vi "Main_Equip_Radiació.vi"() -> ()   [LabVIEW 2017]
uses:
  <vilib>/DAQmx/write.llb/DAQmx Write (Analog DBL 1Chan 1Samp).vi
  <vilib>/DAQmx/write.llb/DAQmx Write (Digital 1D Bool NChan 1Samp 1Line).vi
  <vilib>/DAQmx/read.llb/DAQmx Read (Digital 1D Bool NChan 1Samp 1Line).vi
  <vilib>/DAQmx/miscellaneous.llb/DAQmx Fill In Error Info.vi
panel:
  out "Primera":bool
  out "Factor":dbl
  out "T0":sgl caption="Temperatura" format="%.1f"
  in  "Tipo de Ensayo":enum32{"Calibración", "Ensayo A", "Ensayo B"}(radio)
  out "Nº Tests":u8 caption="Nº pruebas:"
  out "Columna":i32
  out "NMostres":dbl
  out "TablaFinal":dbl[][](array[numeric])
  in  "Consigna  (%)":dbl(slide) min=0.0 max=100.0 scale=0.0..100.0 scale format="%#_3g"
  in  "Poner Pantalla":bool
  in  "Disparo Pantalla":bool
  in  "HORNO":bool
  out "Pantalla retirada":bool
  out "Pantalla colocada":bool
  in  "Dades":dbl[](array[numeric])
  out "hardware name":string
  out "IndexSup":i32
  out "IndexInf":i32
  in  "Verifica":bool
  out "High Time":sgl format="%#_3g"
  out "Low Time":sgl format="%#_3g"
  in  "High Temp.":sgl
  in  "Low Temp.":sgl
  out "Temps":sgl caption="Tiempo" format="%.1f"
  out "Calibration result:":bool
  out "error out_USB":errorcluster
  out "Nom Sensor Temperatura":string
  in  "Guardar 24h":bool caption="Informe"
  out "Dies":u8 caption="NumDies"
  in  "Reset_AutoSave 24":bool
  in  "mT1":sgl caption="Temperatura_1" format="%.1f"
  out "Maxim":sgl
  in  "BtSalir":bool caption="Sortir"
  in  "Reset_AutoSave":bool
  in  "Nombre test:":string
  out "Gràfiques T-Temps":cluster{"Value":sgl[], "Value":sgl[]}[](graph)
  in  "Datos OK":bool
  out "DadesComplertes":sgl[](array[numeric])
  in  "Grafica_OK":bool=TRUE
  out "Tabla":sgl[][](array[numeric])
  in  "Registro OK":bool=TRUE
  in  "time out":bool
  in  "Reset_gráfica":bool
  in  "Reset_Time":bool
  in  "Tiempo_string":string[](array[string])
  out "Elapsed Time (s)":i32
  out "Ensayo activo":bool
  out "FSenseTara":sgl caption="Fuerza - N"
  in  "CaptadorF":u16(ring) caption="Unidades" items=["25kg"=5]
  in  "PendentLlum":sgl caption="Força" format="%.1f"
  out "FactorsUnitatsPendents_F":dbl[](array[numeric])
  out "ConversioUnitatsF":dbl[](array[numeric])=[1.0, 9.8756, 2.2]
  out "ArraiUnitats":cluster{"String":string, "Value":u16}[](array[cluster])=[{"String"="kg", "Value"=0}, {"String"="N", "Value"=1}, {"String"="g", "Value"=2}, {"String"="daN", "Value"=3}, {"String"="cN", "Value"=4}, {"String"="KN", "Value"=5}, {"String"="lb", "Value"=6}]
  out "Tara":sgl caption="Força" format="%.1f"
  out "Temperatura1":sgl caption="Temperatura" format="%.1f"
  out "PendentsT":sgl[](array[numeric])
  in  "Salir":bool caption="Sortir"
  in  "Ensayonuevo":bool caption="New Test"
  in  "Guardar":bool
  in  "Iniciar / Finalizar":bool=TRUE caption="Finalitzar prova"
  in  "UnidadesF":u16(ring) caption="Unidades" items=["kg", "N", "g"]
  in  "BtTaraPot":bool caption="TARA"
  # "sg"
  # "ºC"
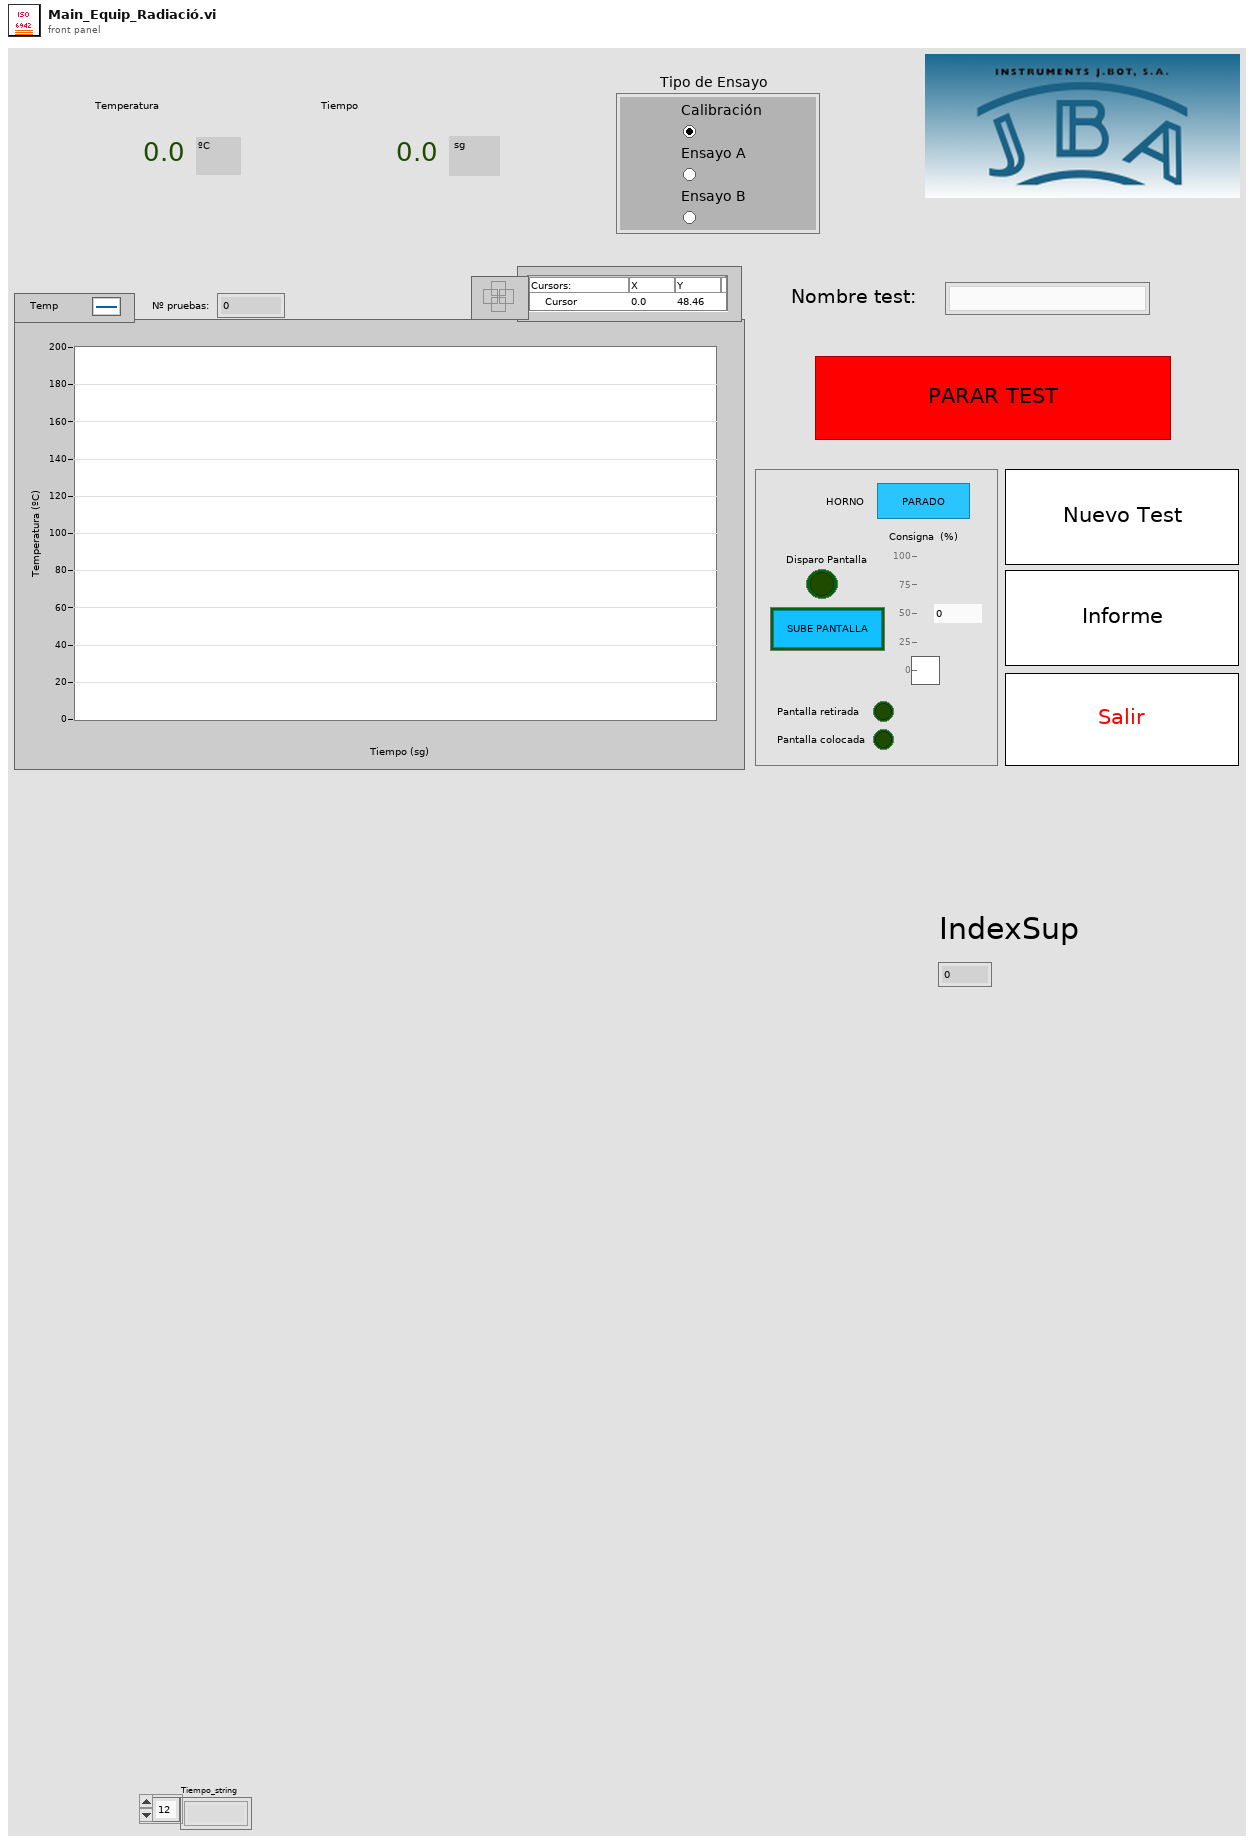
[diagram p1: front panel]
types:
  T1 = enum8{"Enabled", "Disabled", "Disabled and Grayed Out"}
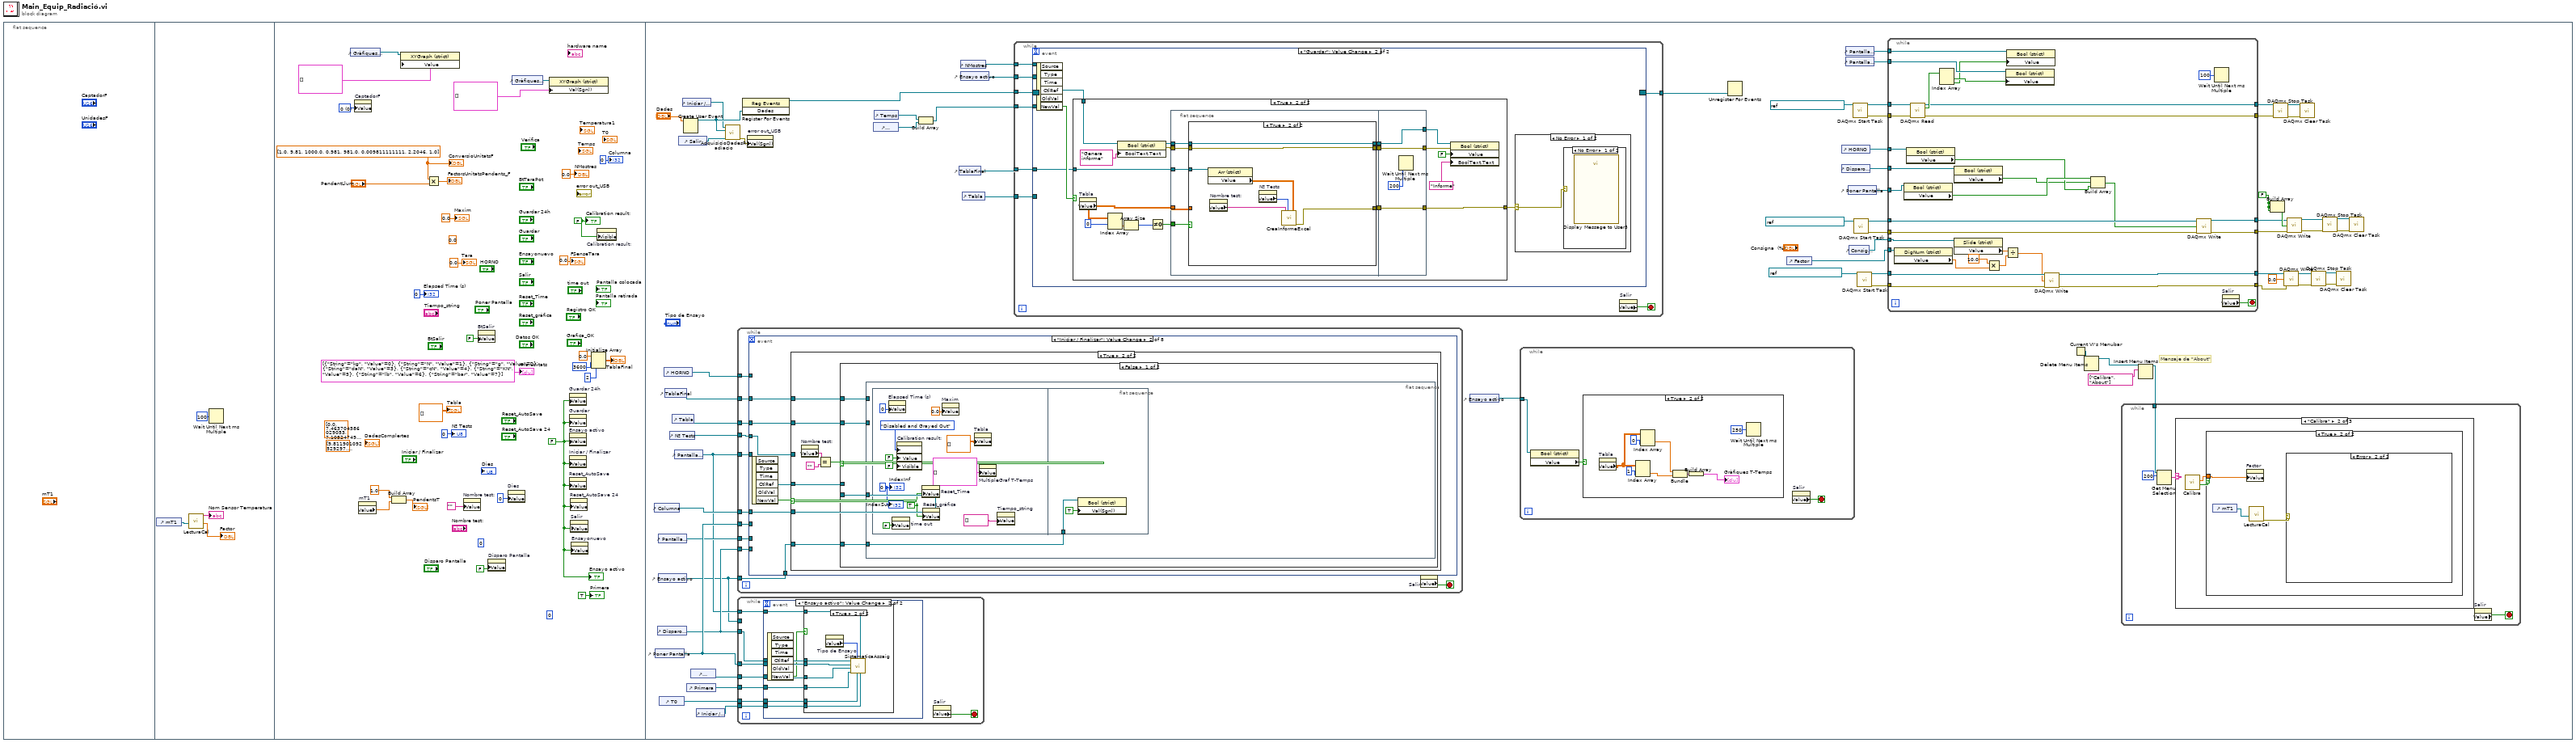
[diagram p0: block diagram]
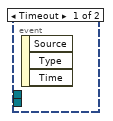
[diagram p2: hidden frame]
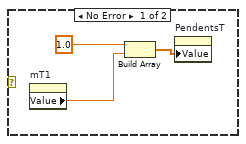
[diagram p6: hidden frame]
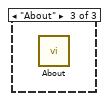
[diagram p7: hidden frame]
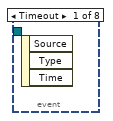
[diagram p9: hidden frame]
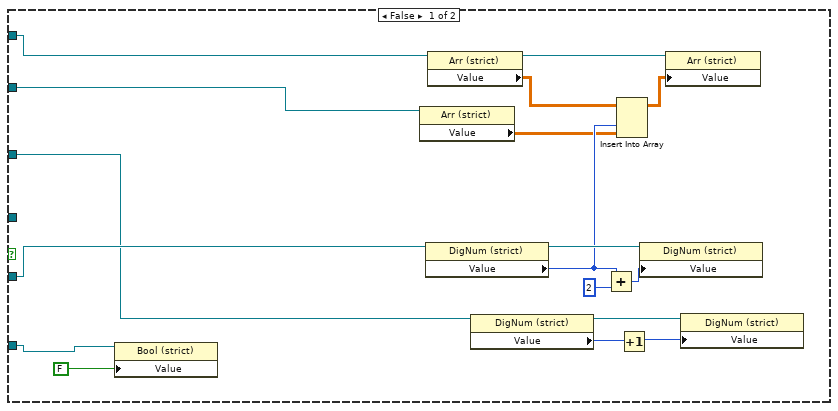
[diagram p10: hidden frame]
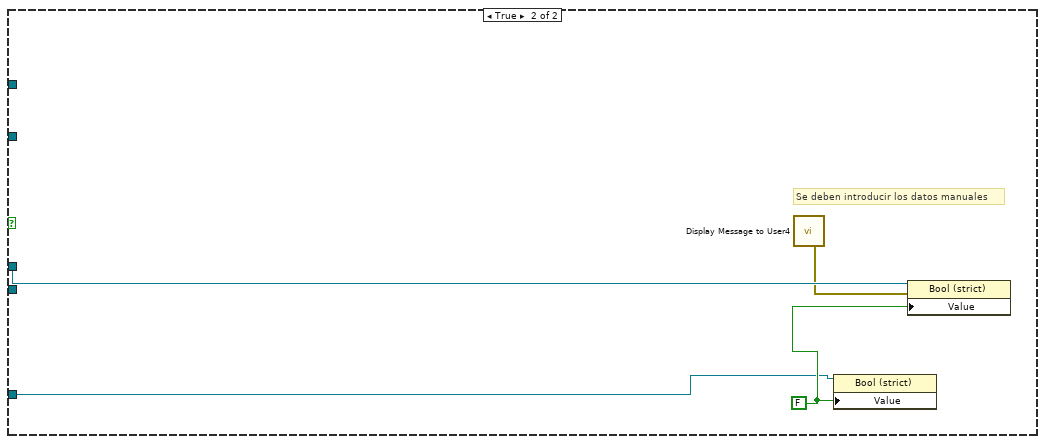
[diagram p11: hidden frame]
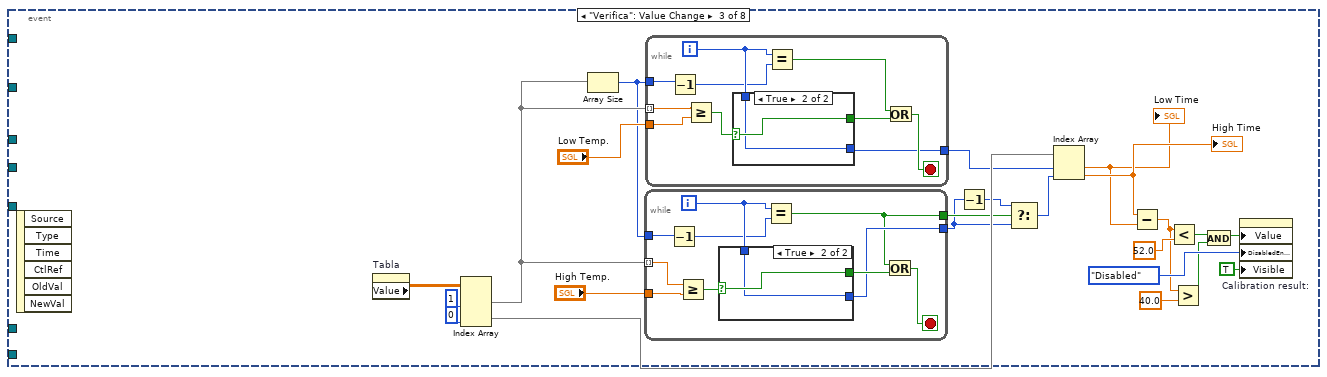
[diagram p12: hidden frame]
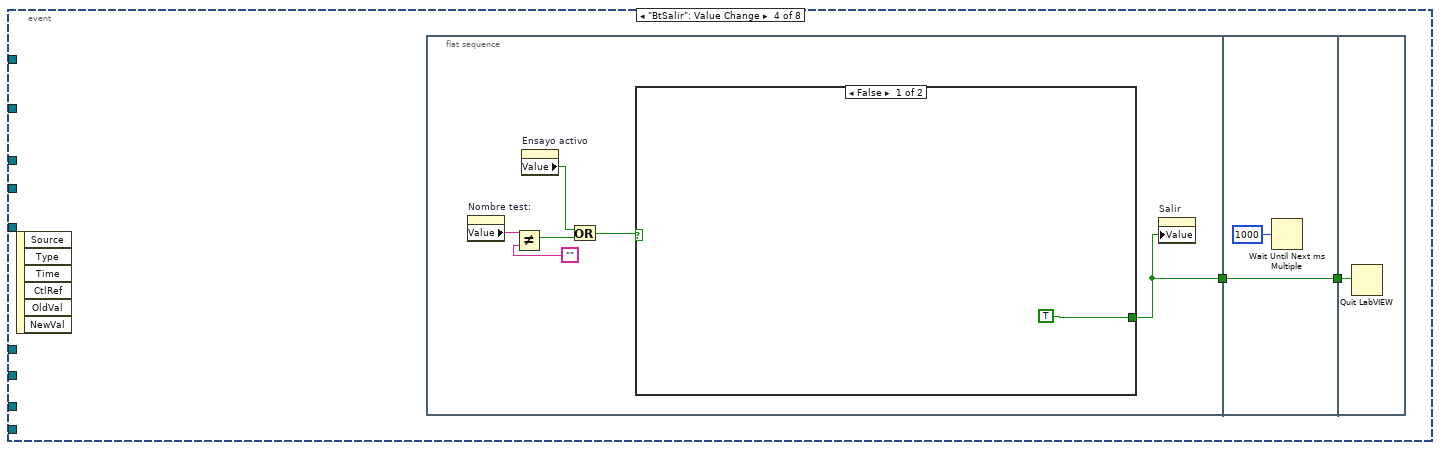
[diagram p15: hidden frame]
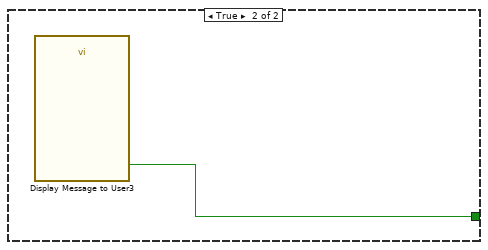
[diagram p16: hidden frame]
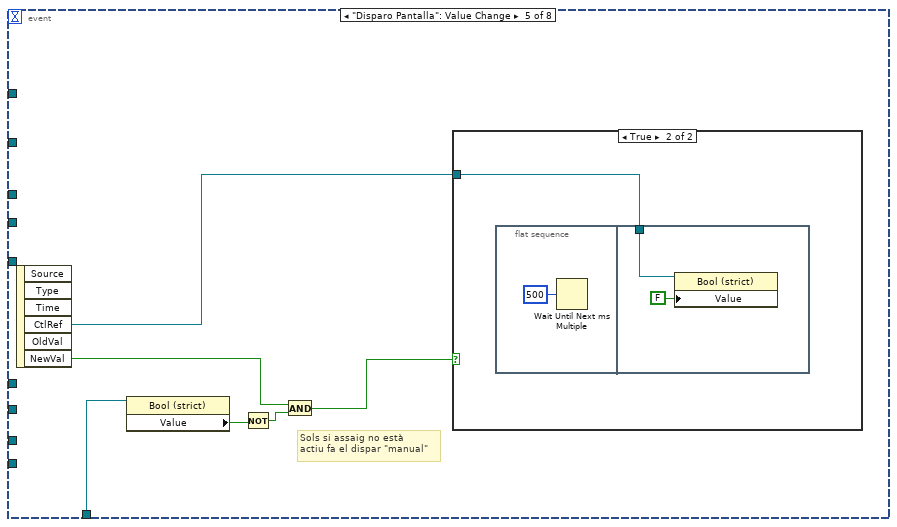
[diagram p17: hidden frame]
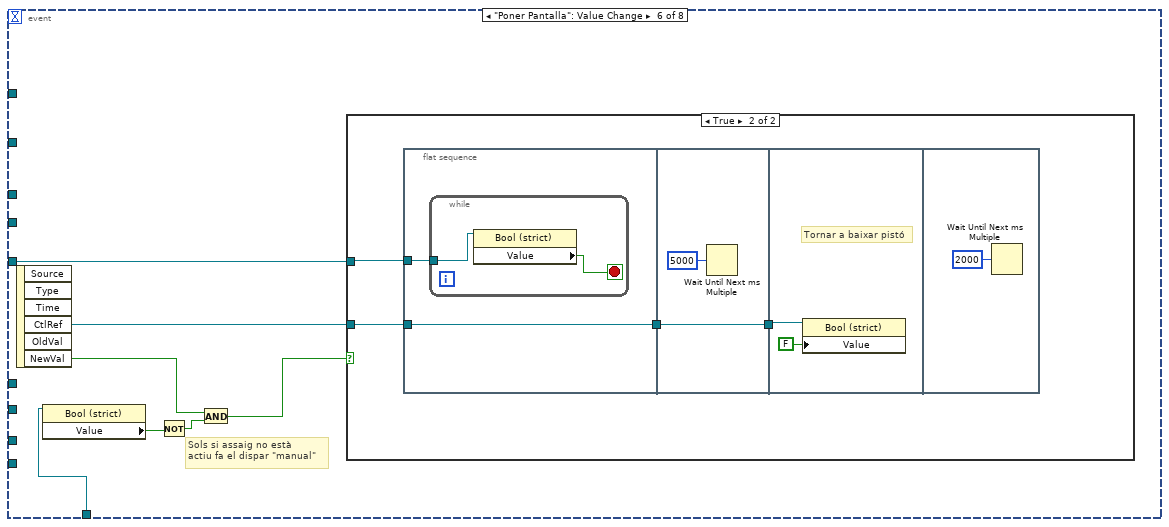
[diagram p19: hidden frame]
diagram:
  n1 = flat-sequence {
    frame #0 {
    }
    frame #1 {
      n2 = control-ref of="mT1"() -> (w2:refnum<vi>)
      n3 = call "LecturaCal.vi"("T1"=w2) -> ("Factor Potència"=→"Factor":dbl, "Nom Sensor Temperatura"=→"Nom Sensor Temperatura":string)  [unwired: 8 in, 1 out]
      n4 = Wait Until Next ms Multiple(millisecond multiple=u32 100) -> ()  [unwired: 1 out]
    }
    frame #2 {
      w18 = FALSE ("Resultat Assaig")
      (unwired) sgl[] [9.811901, 9.763803, 9.671529, 9.535354] ("DadesComplertes")
      (unwired) sgl[][] [[0.0, 7.4637046, 7.1052475, 6.7309566, 6.297442], [5.0, 2.5386999, 2.902987, 3.276568, 3.6958933], [10.0, 7.471229, 7.101099, 6.7181377, 6.2959595], [15.0, 2.5153666, 2.9171765, 3.291629, 3.679636], [20.0, 7.4759755, 7.089289, 6.711311, 6.298526]] ("Tabla")
      (unwired) u8 0 ("Durada assaig minuts")
      (unwired) u8 0 ("Durada assaig - hores:")
      w27 = u16 0 items=["0"] ("CaptadorF")
      (unwired) sgl 0.0 ("Fuerza")
      w6 = FALSE ("Ensayo activo")
      w34 = dbl[] [1.0, 9.81, 1000.0, 0.981, 981.0, 0.009811111111, 2.2046, 1.0]
      n5 = control-ref of="Gràfiques T-Temps"() -> (w20:refnum<vi>)
      n6 = property on="CaptadorF" class="Ring (strict)"("Value"=w27) -> ()  [unwired: 2 in, 2 out]
      n7 = property on="mT1" class="DigNum (strict)"() -> ("Value"=w7:sgl)  [unwired: 2 in, 2 out]
      n8 = Build Array(sgl 1.0 ("element"), w7) -> (→"PendentsT":sgl[])
      n9 = property class="XYGraph (strict)"(reference=w20, "Value"=cluster{"Value":sgl[], "Value":sgl[]}[] []) -> ()  [unwired: 1 in, 2 out]
      n10 = Multiply(x=w34, y="PendentLlum") -> (x*y=→"FactorsUnitatsPendents_F":dbl[])
      n11 = property on="Nombre test:" class="Str"("Value"="") -> ()  [unwired: 2 in, 2 out]
      n12 = property on="BtSalir" class="Bool (strict)"("Value"=FALSE ("BtSalir")) -> ()  [unwired: 2 in, 2 out]
      n13 = property on="Disparo Pantalla" class="Bool (strict)"("Value"=FALSE ("Quitar Pantalla")) -> ()  [unwired: 2 in, 2 out]
      n14 = property on="Dies" class="DigNum (strict)"("Value"=u8 0 ("NumDies")) -> ()  [unwired: 2 in, 2 out]
      n15 = control-ref of="Gràfiques T-Temps"() -> (w23:refnum<vi>)
      n16 = property class="XYGraph (strict)"(reference=w23, "Val(Sgnl)"=cluster{"Value":sgl[], "Value":sgl[]}[] [] ("Value")) -> ()  [unwired: 1 in, 2 out]
      n17 = property on="Guardar 24h" class="Bool (strict)"("Value"=w6) -> ()  [unwired: 2 in, 2 out]
      n18 = property on="Guardar" class="Bool (strict)"("Value"=w6) -> ()  [unwired: 2 in, 2 out]
      n19 = property on="Ensayo activo" class="Bool (strict)"("Value"=w6) -> ()  [unwired: 2 in, 2 out]
      n20 = property on="Iniciar / Finalizar" class="Bool (strict)"("Value"=w6) -> ()  [unwired: 2 in, 2 out]
      n21 = property on="Reset_AutoSave" class="Bool (strict)"("Value"=w6) -> ()  [unwired: 2 in, 2 out]
      n22 = property on="Reset_AutoSave 24" class="Bool (strict)"("Value"=w6) -> ()  [unwired: 2 in, 2 out]
      n23 = property on="Salir" class="Bool (strict)"("Value"=w6) -> ()  [unwired: 2 in, 2 out]
      n24 = property on="Ensayonuevo" class="Bool (strict)"("Value"=w6) -> ()  [unwired: 2 in, 2 out]
      n25 = Initialize Array(0.0 ("element"), 3600 ("dimension size"), 2 ("dimension size")) -> (→"TablaFinal":dbl[][])
      n26 = property on="Calibration result:" class="Bool (strict)"("Visible"=w18) -> ()  [unwired: 2 in, 2 out]
      "Tara" <- sgl 0.0 ("Tara")
      "ArraiUnitats" <- cluster{"String":string, "Value":u16}[] [{"String"="kg", "Value"=0}, {"String"="N", "Value"=1}, {"String"="g", "Value"=2}, {"String"="daN", "Value"=3}, {"String"="cN", "Value"=4}, {"String"="KN", "Value"=5}, {"String"="lb", "Value"=6}, {"String"="bar", "Value"=7}] ("Strings And Values [] 2")
      "ConversioUnitatsF" <- w34
      "FSenseTara" <- sgl 0.0 ("FSenseTara")
      "Elapsed Time (s)" <- 0 ("Elapsed Time (s)")
      "Tabla" <- sgl[][] [] ("Tabla")
      "Maxim" <- sgl 0.0 ("Maxim")
      "Calibration result:" <- w18
      "Ensayo activo" <- w6
      "NMostres" <- 0.0 ("NMostres")
      "Columna" <- 0 ("Columna")
      "Nº Tests" <- u8 0 ("Nº Tests")
      "Primera" <- TRUE ("Primera")
    }
    frame #3 {
      w47 = FALSE ("Value")
      # "Mensaje de \"About\""
      n27 = control-ref of="Columna"() -> (w64:refnum<vi>)
      n28 = control-ref of="Poner Pantalla"() -> (w55:refnum<vi>)
      n29 = control-ref of="Disparo Pantalla"() -> (w53:refnum<vi>)
      n30 = control-ref of="Pantalla retirada"() -> (w54:refnum<vi>)
      n31 = control-ref of="Ensayo activo"() -> (w48:refnum<vi>)
      n32 = control-ref of="T0"() -> (w57:refnum<vi>)
      n33 = control-ref of="HORNO"() -> (w59:refnum<vi>)
      n34 = control-ref of="TablaFinal"() -> (w65:refnum<vi>)
      n35 = control-ref of="Nº Tests"() -> (w62:refnum<vi>)
      n36 = control-ref of="Tabla"() -> (w63:refnum<vi>)
      n37 = control-ref of="Pantalla colocada"() -> (w51:refnum<vi>)
      n38 = control-ref of="Salir"() -> (w93:refnum<vi>)
      n39 = control-ref of="Iniciar / Finalizar"() -> (w89:refnum<vi>)
      n40 = Create User Event(user event datatype="Dades") -> (user event=w90:refnum<user-event>)  [unwired: 1 in, 1 out]
      n41 = control-ref of="Primera"() -> (w36:refnum<vi>)
      n42 = control-ref of="Temperatura1"() -> (w58:refnum<vi>)
      n43 = control-ref of="Iniciar / Finalizar"() -> (w52:refnum<vi>)
      n44 = call "AdquisicioDadesRadiacio.vi"("Stop"=w93, "EventDades"=w90, "AssaigActiu"=w89) -> ("error out"=w92:errorcluster)  [unwired: 8 in]
      n45 = while {
        tunnel: w65 -> [w193]
        tunnel: w64 -> [w192]
        tunnel: w63 -> [w191]
        tunnel: w62 -> [w190]
        tunnel: w59 -> [w189]
        tunnel: w51 -> [w188]
        tunnel: w55 -> [w187]
        tunnel: w54 -> [w186]
        tunnel: w53 -> [w185]
        tunnel: w48 -> [w184]
        stop <- w194 stop-if-true
        n46 = event shown="[1] \"Iniciar / Finalizar\": Value Change" {
          selector: _ -> [_ _ _ _ _ _ _ _]
          dyn-events: _ -> [_ _ _ _ _ _ _ _]
          timeout: _ -> [_ _ _ _ _ _ _ _]
          tunnel: w193 -> [_ w199 _ _ _ _ _ w343]
          tunnel: w192 -> [_ w198 _ _ _ _ _ w341]
          tunnel: w191 -> [_ w197 _ _ _ _ _ _]
          tunnel: w190 -> [_ w196 _ _ _ _ _ w345]
          tunnel: w189 -> [_ _ _ _ _ _ _ _]
          tunnel: w188 -> [_ _ _ _ _ w327 _ _]
          tunnel: w187 -> [_ _ _ _ _ _ _ _]
          tunnel: w186 -> [_ _ _ _ _ _ _ _]
          tunnel: w185 -> [_ _ _ _ _ _ _ _]
          tunnel: w184 -> [_ w195 _ _ w315 w323 _ _]
          event Timeout {
            n47 = event-data() -> ()  [unwired: 1 in, 3 out]
          }
          event "Iniciar / Finalizar": Value Change {
            n48 = event-data() -> ("CtlRef"=w200:refnum<vi>, "NewVal"=w201:bool)  [unwired: 1 in, 4 out]
            n49 = case shown="True" w201 {
              tunnel: w200 -> [_ w226]
              tunnel: w199 -> [w206 w225]
              tunnel: w198 -> [w209 w224]
              tunnel: w197 -> [w207 w223]
              tunnel: w196 -> [w208 _]
              tunnel: w195 -> [w203 w219]
              frame False {
                n50 = property class="Bool (strict)"(reference=w203, "Value"=FALSE ("Ensayo activo")) -> ()  [unwired: 1 in, 2 out]
                n51 = property class="Arr (strict)"(reference=w207) -> ("Value"=w213:sgl[][])  [unwired: 1 in, 2 out]
                n52 = property class="DigNum (strict)"(reference=w209) -> (reference out=w215:refnum<vi>, "Value"=w214:i32)  [unwired: 1 in, 1 out]
                n53 = property class="Arr (strict)"(reference=w206) -> (reference out=w205:refnum<vi>, "Value"=w211:dbl[][])  [unwired: 1 in, 1 out]
                n54 = property on="Property Node" class="DigNum (strict)"(reference=w208) -> (reference out=w204:refnum<vi>, "Value"=w217:u8)  [unwired: 1 in, 1 out]
                n55 = Add(x=w214, y=2) -> (x+y=w216:i32)
                n56 = Insert Into Array(array=w211, index (col)=w214, new element=w213) -> (w212:dbl[][])  [unwired: 1 in]
                n57 = Increment(x=w217) -> (x+1=w218:u8)
                n58 = property class="DigNum (strict)"(reference=w215, "Value"=w216) -> ()  [unwired: 1 in, 2 out]
                n59 = property class="Arr (strict)"(reference=w205, "Value"=w212) -> ()  [unwired: 1 in, 2 out]
                n60 = property on="Property Node" class="DigNum (strict)"(reference=w204, "Value"=w218) -> ()  [unwired: 1 in, 2 out]
              }
              frame True {
                n61 = property on="Nombre test:" class="Str"() -> ("Value"=w222:string)  [unwired: 2 in, 2 out]
                n62 = Equal?(x=w222, y="") -> (x = y?=w220:bool)
                n63 = case shown="False" w220 {
                  tunnel: w226 -> [_ w248]
                  tunnel: w225 -> [w230 _]
                  tunnel: w224 -> [w229 _]
                  tunnel: w223 -> [w228 _]
                  tunnel: w219 -> [w227 w245]
                  frame False {
                    n64 = flat-sequence {
                      tunnel: w228 -> [_]
                      tunnel: w229 -> [_]
                      tunnel: w230 -> [_]
                      tunnel: w227 -> [w231]
                      frame #0 {
                        n65 = flat-sequence {
                          tunnel: w231 -> [w244]
                          frame #0 {
                            w232 = 0 ("IndexInf")
                            w240 = TRUE ("Reset_Time")
                            n66 = property on="Elapsed Time (s)" class="DigNum (strict)"("Value"=0 ("Elapsed Time (s)")) -> ()  [unwired: 2 in, 2 out]
                            n67 = property on="time out" class="Bool (strict)"("Value"=FALSE ("time out")) -> ()  [unwired: 2 in, 2 out]
                            n68 = property on="Calibration result:" class="Bool (strict)"("DisabledEnum"=T1."Disabled and Grayed Out" ("Disabled"), "Value"=FALSE ("Resultat Assaig"), "Visible"=FALSE) -> ()  [unwired: 2 in, 2 out]
                            n69 = property on="Reset_Time" class="Bool (strict)"("Value"=w240) -> ()  [unwired: 2 in, 2 out]
                            n70 = property on="Reset_gráfica" class="Bool (strict)"("Value"=w240) -> ()  [unwired: 2 in, 2 out]
                            n71 = property on="Maxim" class="DigNum (strict)"("Value"=sgl 0.0 ("Maxim")) -> ()  [unwired: 2 in, 2 out]
                            n72 = property on="Tabla" class="Arr (strict)"("Value"=sgl[][] [] ("Tabla")) -> ()  [unwired: 2 in, 2 out]
                            n73 = property on="MultipleGraf T-Temps" class="XYGraph (strict)"("Value"=cluster{"Y":dbl[], "Y":dbl[]}[] []) -> ()  [unwired: 2 in, 2 out]
                            n74 = property on="Tiempo_string" class="Arr (strict)"("Value"=string[] [] ("Tiempo_string")) -> ()  [unwired: 2 in, 2 out]
                            "IndexSup" <- w232
                            "IndexInf" <- w232
                          }
                          frame #1 {
                            n75 = property class="Bool (strict)"(reference=w244, "Val(Sgnl)"=TRUE ("Iniciar assaig")) -> ()  [unwired: 1 in, 2 out]
                          }
                        }
                      }
                    }
                  }
                  frame True {
                    w246 = FALSE
                    # "Se deben introducir los datos manuales"
                    n76 = call "Display Message to User4"() -> ("error out"=w247:errorcluster)  [unwired: 10 in, 1 out]
                    n77 = property class="Bool (strict)"(reference=w245, "Value"=w246) -> ()  [unwired: 1 in, 2 out]
                    n78 = property class="Bool (strict)"(reference=w248, error in=w247, "Value"=w246) -> ()  [unwired: 2 out]
                  }
                }
              }
            }
          }
          event "Verifica": Value Change {
            n79 = event-data() -> ()  [unwired: 1 in, 6 out]
            n80 = property on="Tabla" class="Arr (strict)"() -> ("Value"=w271:sgl[][])  [unwired: 2 in, 2 out]
            n81 = Index Array(array=w271, index (col) #1=1 ("index (row)"), index (col) #2=0 ("index (row)")) -> (element #1=w262:sgl[], element #2=w259:sgl[])  [unwired: 2 in]
            n82 = Array Size(array=w262) -> (size(s)=w260:i32)
            n83 = while {
              tunnel: w262 -> [w281] mode=indexing
              tunnel: "High Temp." -> [w275]
              tunnel: w260 -> [w274]
              tunnel: [w273] -> w249
              tunnel: [w272] -> w252
              i -> [w279]
              stop <- w276 stop-if-true
              n84 = Decrement(x=w274) -> (x-1=w278:i32)
              n85 = Greater Or Equal?(x=w281, y=w275) -> (x >= y?=w280:bool)
              n86 = case shown="True" w280 {
                selector: w280 -> [w282 w284]
                tunnel: w279 -> [_ w283]
                tunnel: [w282 w284] -> w277
                tunnel: [_ w283] -> w273
                frame False {
                }
                frame True {
                }
              }
              n87 = Equal?(x=w279, y=w278) -> (x = y?=w272:bool)
              n88 = Or(x=w272, y=w277) -> (x .or. y?=w276:bool)
            }
            n89 = while {
              tunnel: w262 -> [w294] mode=indexing
              tunnel: "Low Temp." -> [w293]
              tunnel: w260 -> [w290]
              tunnel: [w285] -> w258
              i -> [w291]
              stop <- w286 stop-if-true
              n90 = Decrement(x=w290) -> (x-1=w289:i32)
              n91 = Greater Or Equal?(x=w294, y=w293) -> (x >= y?=w292:bool)
              n92 = case shown="True" w292 {
                selector: w292 -> [w295 w297]
                tunnel: w291 -> [_ w296]
                tunnel: [w295 w297] -> w287
                tunnel: [_ w296] -> w285
                frame False {
                }
                frame True {
                }
              }
              n93 = Equal?(x=w291, y=w289) -> (x = y?=w288:bool)
              n94 = Or(x=w288, y=w287) -> (x .or. y?=w286:bool)
            }
            n95 = Decrement(x=w249) -> (x-1=w250:i32)
            n96 = Select(t=w250, s=w252, f=w249) -> (s? t:f=w251:i32)
            n97 = Index Array(array=w259, index #1=w258, index #2=w251) -> (element #1=w266:sgl, element #2=w267:sgl)
            "Low Time" <- w266
            "High Time" <- w267
            n98 = Subtract(x=w267, y=w266) -> (x-y=w256:sgl)
            n99 = Less?(x=w256, y=sgl 52.0) -> (x < y?=w254:bool)
            n100 = Greater?(x=w256, y=40.0) -> (0:w253:bool)
            n101 = And(x=w254, y=w253) -> (x .and. y?=w255:bool)
            n102 = property on="Calibration result:" class="Bool (strict)"("Value"=w255, "DisabledEnum"=T1."Disabled" ("Disabled"), "Visible"=TRUE) -> ()  [unwired: 2 in, 2 out]
          }
          event "BtSalir": Value Change {
            n103 = event-data() -> ()  [unwired: 1 in, 6 out]
            n104 = flat-sequence {
              tunnel: [w305] -> w299
              tunnel: w299 -> [w309]
              tunnel: [w309] -> w298
              tunnel: w298 -> [w310]
              frame #0 {
                n105 = property on="Nombre test:" class="Str"() -> ("Value"=w304:string)  [unwired: 2 in, 2 out]
                n106 = Not Equal?(x=w304, y="") -> (x != y?=w300:bool)
                n107 = property on="Ensayo activo" class="Bool (strict)"() -> ("Value"=w301:bool)  [unwired: 2 in, 2 out]
                n108 = Or(x=w301, y=w300) -> (x .or. y?=w302:bool)
                n109 = case shown="False" w302 {
                  tunnel: [TRUE ("OK") w307] -> w305
                  frame False {
                  }
                  frame True {
                    n110 = call "Display Message to User3"() -> ("OK"=w307:bool)  [unwired: 10 in, 1 out]
                  }
                }
                n111 = property on="Salir" class="Bool (strict)"("Value"=w305) -> ()  [unwired: 2 in, 2 out]
              }
              frame #1 {
                n112 = Wait Until Next ms Multiple(millisecond multiple=u32 1000) -> ()  [unwired: 1 out]
              }
              frame #2 {
                n113 = Quit LabVIEW(quit? (T)=w310) -> ()
              }
            }
          }
          event "Disparo Pantalla": Value Change {
            # "Sols si assaig no està\nactiu fa el dispar \"manual\""
            n114 = event-data() -> ("CtlRef"=w316:refnum<vi>, "NewVal"=w312:bool)  [unwired: 1 in, 4 out]
            n115 = property class="Bool (strict)"(reference=w315) -> ("Value"=w314:bool)  [unwired: 1 in, 2 out]
            n116 = Not(x=w314) -> (.not. x?=w313:bool)
            n117 = And(x=w312, y=w313) -> (x .and. y?=w311:bool)
            n118 = case shown="True" w311 {
              tunnel: w316 -> [_ w317]
              frame False {
              }
              frame True {
                n119 = flat-sequence {
                  tunnel: w317 -> [w320]
                  frame #0 {
                    n120 = Wait Until Next ms Multiple(millisecond multiple=u32 500) -> ()  [unwired: 1 out]
                  }
                  frame #1 {
                    n121 = property class="Bool (strict)"(reference=w320, "Value"=FALSE) -> ()  [unwired: 1 in, 2 out]
                  }
                }
              }
            }
          }
          event "Poner Pantalla": Value Change {
            # "Sols si assaig no està\nactiu fa el dispar \"manual\""
            n122 = event-data() -> ("CtlRef"=w326:refnum<vi>, "NewVal"=w322:bool)  [unwired: 1 in, 4 out]
            n123 = property class="Bool (strict)"(reference=w323) -> ("Value"=w325:bool)  [unwired: 1 in, 2 out]
            n124 = Not(x=w325) -> (.not. x?=w324:bool)
            n125 = And(x=w322, y=w324) -> (x .and. y?=w321:bool)
            n126 = case shown="True" w321 {
              tunnel: w327 -> [_ w331]
              tunnel: w326 -> [_ w330]
              frame False {
              }
              frame True {
                n127 = flat-sequence {
                  tunnel: w331 -> [w333]
                  tunnel: w330 -> [w332]
                  tunnel: [w332] -> w329
                  tunnel: w329 -> [w336]
                  tunnel: [w336] -> w328
                  tunnel: w328 -> [w339]
                  frame #0 {
                    n128 = while {
                      tunnel: w333 -> [w335]
                      stop <- w334 stop-if-true
                      n129 = property class="Bool (strict)"(reference=w335) -> ("Value"=w334:bool)  [unwired: 1 in, 2 out]
                    }
                  }
                  frame #1 {
                    n130 = Wait Until Next ms Multiple(millisecond multiple=u32 5000) -> ()  [unwired: 1 out]
                  }
                  frame #2 {
                    # "Tornar a baixar pistó"
                    n131 = property class="Bool (strict)"(reference=w339, "Value"=FALSE) -> ()  [unwired: 1 in, 2 out]
                  }
                  frame #3 {
                    n132 = Wait Until Next ms Multiple(millisecond multiple=u32 2000) -> ()  [unwired: 1 out]
                  }
                }
              }
            }
          }
          event "error out_USB": Value Change {
            n133 = event-data() -> ()  [unwired: 1 in, 6 out]
            n134 = call "Display Message to User10"() -> ()  [unwired: 10 in, 2 out]
          }
          event "Ensayonuevo": Value Change {
            n135 = event-data() -> ("CtlRef"=w349:refnum<vi>, "NewVal"=w346:bool)  [unwired: 1 in, 4 out]
            n136 = property class="DigNum (strict)"(reference=w345) -> (reference out=w342:refnum<vi>, "Value"=w344:u8)  [unwired: 1 in, 1 out]
            n137 = Not Equal To 0?(x=w344) -> (x != 0?=w347:bool)
            n138 = And(x=w347, y=w346) -> (x .and. y?=w348:bool)
            n139 = case shown="True" w348 {
              tunnel: w349 -> [w353 w358]
              tunnel: [w353 w358] -> w350
              tunnel: [FALSE ("Value") FALSE ("Value")] -> w351
              tunnel: w343 -> [_ w356]
              tunnel: w342 -> [_ w355]
              tunnel: w341 -> [_ w354]
              frame False {
              }
              frame True {
                n140 = call "Display Message to User6"() -> ("Yes"=w359:bool)  [unwired: 10 in, 1 out]
                n141 = case shown="True" w359 {
                  tunnel: w356 -> [_ w366]
                  tunnel: w355 -> [_ w364]
                  tunnel: w354 -> [_ w362]
                  frame False {
                  }
                  frame True {
                    (unwired) "00:00:00" ("Tiempo transcurrido (hh:mm:ss)")
                    w371 = TRUE ("Reset_Time")
                    (unwired) cluster{"Value":sgl[], "Value":sgl[]} {"Value"=[], "Value"=[]} ("Grafica F-T")
                    n142 = property class="DigNum (strict)"(reference=w362, "Value"=0) -> ()  [unwired: 1 in, 2 out]
                    n143 = property class="Arr (strict)"(reference=w366, "Value"=dbl[][] []) -> ()  [unwired: 1 in, 2 out]
                    n144 = property class="DigNum (strict)"(reference=w364, "Value"=u8 0) -> ()  [unwired: 1 in, 2 out]
                    n145 = property on="Reset_Time" class="Bool (strict)"("Value"=w371) -> ()  [unwired: 2 in, 2 out]
                    n146 = property on="Reset_gráfica" class="Bool (strict)"("Value"=w371) -> ()  [unwired: 2 in, 2 out]
                    n147 = property on="Tiempo_string" class="Arr (strict)"("Value"=string[] [] ("Tiempo_string")) -> ()  [unwired: 2 in, 2 out]
                    n148 = property on="Nombre test:" class="Str"("Value"="") -> ()  [unwired: 2 in, 2 out]
                    n149 = property on="Tabla" class="Arr (strict)"("Value"=sgl[][] [] ("Tabla")) -> ()  [unwired: 2 in, 2 out]
                    n150 = property on="Gràfiques T-Temps" class="XYGraph (strict)"("Value"=cluster{"Y":dbl[], "Y":dbl[]}[] []) -> ()  [unwired: 2 in, 2 out]
                    n151 = property on="Primera" class="Bool (strict)"("Value"=TRUE ("Primera")) -> ()  [unwired: 2 in, 2 out]
                    n152 = property on="Elapsed Time (s)" class="DigNum (strict)"("Value"=0 ("Elapsed Time (s)")) -> ()  [unwired: 2 in, 2 out]
                    n153 = property on="time out" class="Bool (strict)"("Value"=FALSE ("time out")) -> ()  [unwired: 2 in, 2 out]
                    n154 = property on="Maxim" class="DigNum (strict)"("Value"=sgl 0.0 ("Maxim")) -> ()  [unwired: 2 in, 2 out]
                  }
                }
              }
            }
            n155 = property class="Bool (strict)"(reference=w350, "Value"=w351) -> ()  [unwired: 1 in, 2 out]
          }
        }
        n156 = property on="Salir" class="Bool (strict)"() -> ("Value"=w194:bool)  [unwired: 2 in, 2 out]
      }
      n157 = while {
        tunnel: w58 -> [w111]
        tunnel: w57 -> [w110]
        tunnel: w53 -> [w109]
        tunnel: w55 -> [w108]
        tunnel: w48 -> [_]
        tunnel: w52 -> [w106]
        tunnel: w51 -> [w105]
        tunnel: w36 -> [w104]
        stop <- w107 stop-if-true
        n158 = event shown="[1] \"Ensayo activo\": Value Change" {
          selector: _ -> [_ _]
          dyn-events: _ -> [_ _]
          timeout: _ -> [_ _]
          tunnel: w111 -> [_ w119]
          tunnel: w110 -> [_ w118]
          tunnel: w109 -> [_ w117]
          tunnel: w108 -> [_ w116]
          tunnel: w106 -> [_ w115]
          tunnel: w105 -> [_ w114]
          tunnel: w104 -> [_ w113]
          event Timeout {
            n159 = event-data() -> ()  [unwired: 1 in, 3 out]
          }
          event "Ensayo activo": Value Change {
            n160 = event-data() -> ("NewVal"=w112:bool)  [unwired: 1 in, 5 out]
            n161 = case shown="True" w112 {
              tunnel: w119 -> [_ w126]
              tunnel: w118 -> [_ w125]
              tunnel: w117 -> [_ w124]
              tunnel: w116 -> [_ w123]
              tunnel: w115 -> [_ w122]
              tunnel: w114 -> [_ w121]
              tunnel: w113 -> [_ w120]
              frame False {
              }
              frame True {
                n162 = property on="Tipo de Ensayo" class="RadioBtnsControl (strict)"() -> ("Value"=w127:enum32{"Calibración", "Ensayo A", "Ensayo B"})  [unwired: 2 in, 2 out]
                n163 = call "SistematicaAssaig.vi"("Iniciar/Finalitzar"=w122, "PantallaColocada"=w121, "T0"=w125, "Value"=w127, "Primera"=w120, "Temperatura1"=w126, "Poner Pantalla"=w123, "DisparoPantalla"=w124) -> ()  [unwired: 4 in]
              }
            }
          }
        }
        n164 = property on="Salir" class="Bool (strict)"() -> ("Value"=w107:bool)  [unwired: 2 in, 2 out]
      }
      n165 = register-events(w90) -> (reference out=w102:refnum<event-registration>)  [unwired: 2 in, 1 out]
      n166 = property on="error out_USB" class="Clust (strict)"("Val(Sgnl)"=w92) -> ()  [unwired: 2 in, 2 out]
      n167 = control-ref of="Temperatura1"() -> (w94:refnum<vi>)
      n168 = control-ref of="Temps"() -> (w95:refnum<vi>)
      n169 = Build Array(w95, w94) -> (w97:refnum<vi>[])
      n170 = control-ref of="TablaFinal"() -> (w61:refnum<vi>)
      n171 = control-ref of="NMostres"() -> (w66:refnum<vi>)
      n172 = control-ref of="Ensayo activo"() -> (w96:refnum<vi>)
      n173 = control-ref of="Tabla"() -> (w60:refnum<vi>)
      n174 = while {
        tunnel: w102 -> [w382]
        tunnel: [w381] -> w103
        tunnel: w97 -> [w379]
        tunnel: w96 -> [w378]
        tunnel: w66 -> [w377]
        tunnel: w61 -> [w376]
        tunnel: w60 -> [w375]
        stop <- w380 stop-if-true
        n175 = event shown="[1] \"Guardar\": Value Change" {
          selector: w382 -> [_ _]
          dyn-events: [_ _] -> w381
          timeout: _ -> [_ _]
          tunnel: w379 -> [w389 _]
          tunnel: w378 -> [w388 _]
          tunnel: w377 -> [w384 _]
          tunnel: w376 -> [_ w404]
          tunnel: w375 -> [w383 _]
          event User Event {
            n176 = event-data() -> ("Dades"=w385:dbl[])  [unwired: 1 in, 4 out]
            n177 = property on="PendentsT" class="Arr (strict)"() -> ("Value"=w390:sgl[])  [unwired: 2 in, 2 out]
            n178 = Multiply(x=w385, y=w390) -> (x*y=w386:dbl[])
            n179 = for {
              tunnel: w389 -> [w392] mode=indexing
              tunnel: w386 -> [w393] mode=indexing
              # "Precisió 2 i 1"
              n180 = property class="DigNum (strict)"(reference=w392, "Value"=w393, "Precision"=u8 1 ("Display Format:Precision")) -> ()  [unwired: 1 in, 2 out]
            }
            n181 = property class="Bool (strict)"(reference=w388) -> ("Value"=w387:bool)  [unwired: 1 in, 2 out]
            n182 = case shown="True" w387 {
              tunnel: w386 -> [_ w394]
              tunnel: w384 -> [_ w403]
              tunnel: w383 -> [_ w398]
              frame False {
              }
              frame True {
                n183 = property class="DigNum (strict)"(reference=w403) -> (reference out=w402:refnum<vi>, error out=w401:errorcluster, "Value"=w400:dbl)  [unwired: 1 in]
                n184 = property class="Arr (strict)"(reference=w398) -> (reference out=w397:refnum<vi>, "Value"=w396:sgl[][])  [unwired: 1 in, 1 out]
                n185 = Build Array (concatenate)(w396, w394) -> (w395:dbl[][])
                n186 = Increment(x=w400) -> (x+1=w399:dbl)
                n187 = property class="DigNum (strict)"(reference=w402, error in=w401, "Value"=w399) -> ()  [unwired: 2 out]
                n188 = property class="Arr (strict)"(reference=w397, "Value"=w395) -> ()  [unwired: 1 in, 2 out]
              }
            }
          }
          event "Guardar": Value Change {
            n189 = event-data() -> ("CtlRef"=w405:refnum<vi>, "NewVal"=w407:bool)  [unwired: 1 in, 4 out]
            n190 = case shown="True" w407 {
              tunnel: [errorcluster {"status"=FALSE, "code"=0, "source"=""} ("error out") w428] -> w406
              tunnel: w405 -> [_ w418]
              tunnel: w404 -> [_ w411]
              frame False {
              }
              frame True {
                n191 = property on="Tabla" class="Arr (strict)"() -> ("Value"=w412:sgl[][])  [unwired: 2 in, 2 out]
                n192 = Index Array(array=w412, index (row)=0) -> (element=w426:sgl[])  [unwired: 1 in]
                n193 = property class="Bool (strict)"(reference=w418, "BoolText.Text"="Genera informe" ("Boolean Text.Text")) -> (reference out=w417:refnum<vi>, error out=w413:errorcluster)  [unwired: 1 in]
                n194 = Array Size(array=w426) -> (size(s)=w414:i32)
                n195 = Not Equal To 0?(x=w414) -> (x != 0?=w425:bool)
                n196 = flat-sequence {
                  tunnel: w412 -> [w435]
                  tunnel: w425 -> [w434]
                  tunnel: w417 -> [w432]
                  tunnel: [w436] -> w421
                  tunnel: [w433] -> w420
                  tunnel: [w431] -> w419
                  tunnel: w413 -> [w430]
                  tunnel: w411 -> [w429]
                  tunnel: [w448] -> w423
                  tunnel: [w449] -> w424
                  tunnel: [w450] -> w428
                  tunnel: w421 -> [w450]
                  tunnel: w420 -> [w449]
                  tunnel: w419 -> [w448]
                  frame #0 {
                    n197 = case shown="True" w434 {
                      tunnel: [errorcluster {"status"=TRUE, "code"=0, "source"=""} ("error out") w444] -> w436
                      tunnel: w435 -> [_ _]
                      tunnel: [w438 w443] -> w433
                      tunnel: w432 -> [w437 w446]
                      tunnel: [w437 w446] -> w431
                      tunnel: w430 -> [_ w443]
                      tunnel: w429 -> [_ w440]
                      frame False {
                        n198 = call "Display Message to User8"() -> ("error out"=w438:errorcluster)  [unwired: 10 in, 1 out]
                      }
                      frame True {
                        n199 = property class="Arr (strict)"(reference=w440) -> ("Value"=w442:dbl[][])  [unwired: 1 in, 2 out]
                        n200 = property on="Nombre test:" class="Str"() -> ("Value"=w445:string)  [unwired: 2 in, 2 out]
                        n201 = property on="Nº Tests" class="DigNum (strict)"() -> ("Value"=w441:u8)  [unwired: 2 in, 2 out]
                        n202 = call "CreaInformeExcel.vi"("Nom Assaig"=w445, "NºTests"=w441, "Tabla"=w442) -> ("error out"=w444:errorcluster)  [unwired: 15 in, 1 out]
                      }
                    }
                  }
                  frame #1 {
                    n203 = Wait Until Next ms Multiple(millisecond multiple=u32 200 ("milliseconds to wait")) -> ()  [unwired: 1 out]
                  }
                }
                n204 = property class="Bool (strict)"(reference=w423, error in=w424, "Value"=FALSE, "BoolText.Text"="Informe" ("Boolean Text.Text")) -> ()  [unwired: 2 out]
              }
            }
            n205 = case shown="No Error" w406 {
              selector: w406 -> [w408 _]
              frame No Error {
                n206 = case shown="No Error" w408 {
                  frame No Error {
                    n207 = call "Display Message to User5"() -> ()  [unwired: 10 in, 2 out]
                  }
                  frame Error {
                    n208 = property on="Reset_AutoSave" class="Bool (strict)"("Value"=FALSE ("Reset_AutoSave")) -> ()  [unwired: 2 in, 2 out]
                  }
                }
              }
              frame Error {
              }
            }
          }
        }
        n209 = property on="Salir" class="Bool (strict)"() -> ("Value"=w380:bool)  [unwired: 2 in, 2 out]
      }
      n210 = control-ref of="Ensayo activo"() -> (w56:refnum<vi>)
      n211 = while {
        tunnel: w56 -> [w174]
        stop <- w175 stop-if-true
        n212 = property class="Bool (strict)"(reference=w174) -> ("Value"=w173:bool)  [unwired: 1 in, 2 out]
        n213 = case shown="True" w173 {
          frame False {
          }
          frame True {
            n214 = property on="Tabla" class="Arr (strict)"() -> ("Value"=w179:sgl[][])  [unwired: 2 in, 2 out]
            n215 = Index Array(array=w179, index (col)=1 ("index")) -> (element=w178:sgl[])  [unwired: 1 in]
            n216 = Index Array(array=w179, index (col)=0 ("index (row)")) -> (element=w177:sgl[])  [unwired: 1 in]
            n217 = Bundle("Value"=w177, "Value"=w178) -> (w183:cluster{"Value":sgl[], "Value":sgl[]})  [unwired: 1 in]
            n218 = Build Array(w183) -> (→"Gràfiques T-Temps":cluster{"Value":sgl[], "Value":sgl[]}[])
            n219 = Wait Until Next ms Multiple(millisecond multiple=u32 250) -> ()  [unwired: 1 out]
          }
        }
        n220 = property on="Salir" class="Bool (strict)"() -> ("Value"=w175:bool)  [unwired: 2 in, 2 out]
      }
      n221 = Unregister For Events(event registration refnum=w103) -> ()  [unwired: 1 in, 1 out]
      n222 = control-ref of="Factor"() -> (w50:refnum<vi>)
      n223 = control-ref of="HORNO"() -> (w76:refnum<vi>)
      n224 = control-ref of="Disparo Pantalla"() -> (w75:refnum<vi>)
      n225 = control-ref of="Pantalla colocada"() -> (w81:refnum<vi>)
      n226 = control-ref of="Pantalla retirada"() -> (w80:refnum<vi>)
      n227 = control-ref of="Poner Pantalla"() -> (w74:refnum<vi>)
      n228 = control-ref of="Consigna  (%)"() -> (w71:refnum<vi>)
      n229 = call <vilib>:"DAQmx Start Task.vi"("task/channels in"=refnum<k21> "USB_Equip_Radiacio_DIn") -> ("task out"=w86:refnum<k21>, "error out"=w70:errorcluster)  [unwired: 13 in]
      n230 = call <vilib>:"DAQmx Start Task.vi"("task/channels in"=refnum<k21> "USB_Equip_Radiacio_DOut") -> ("task out"=w85:refnum<k21>, "error out"=w49:errorcluster)  [unwired: 13 in]
      n231 = call <vilib>:"DAQmx Start Task.vi"("task/channels in"=refnum<k21> "USB_Equip_Radiacio_AO") -> ("task out"=w72:refnum<k21>, "error out"=w69:errorcluster)  [unwired: 13 in]
      n232 = while {
        tunnel: w86 -> [w159]
        tunnel: w85 -> [w154]
        tunnel: [w157] -> w84
        tunnel: w81 -> [w156]
        tunnel: w80 -> [w155]
        tunnel: [w153] -> w44
        tunnel: [w152] -> w77
        tunnel: [w151] -> w43
        tunnel: w76 -> [w150]
        tunnel: w75 -> [w149]
        tunnel: w74 -> [w148]
        tunnel: w72 -> [w147]
        tunnel: w71 -> [w146]
        tunnel: w70 -> [w145]
        tunnel: w69 -> [w144]
        tunnel: [w143] -> w40
        tunnel: [w142] -> w39
        tunnel: w50 -> [w131]
        tunnel: w49 -> [w129]
        stop <- w160 stop-if-true
        n233 = property class="DigNum (strict)"(reference=w131) -> ("Value"=w130:dbl)  [unwired: 1 in, 2 out]
        n234 = property class="Bool (strict)"(reference=w148) -> ("Value"=w141:bool)  [unwired: 1 in, 2 out]
        n235 = property class="Bool (strict)"(reference=w150) -> ("Value"=w136:bool)  [unwired: 1 in, 2 out]
        n236 = call-poly <vilib>:"DAQmx Read.vi"("task/channels in"=w159, "error in"=w145) -> ("task out"=w157:refnum<k21>, "data"=w158:bool[], "error out"=w152:errorcluster)  [unwired: 11 in]
        n237 = Index Array(array=w158) -> (element #1=w140:bool, element #2=w139:bool)  [unwired: 2 in]
        n238 = property class="Bool (strict)"(reference=w149) -> ("Value"=w134:bool)  [unwired: 1 in, 2 out]
        n239 = property class="Slide (strict)"(reference=w146) -> ("Value"=w138:dbl)  [unwired: 1 in, 2 out]
        n240 = Multiply(x=10.0 ("y"), y=w130) -> (x*y=w132:dbl)
        n241 = Divide(x=w138, y=w132) -> (x/y=w137:dbl)
        n242 = property class="Bool (strict)"(reference=w155, "Value"=w140) -> ()  [unwired: 1 in, 2 out]
        n243 = property class="Bool (strict)"(reference=w156, "Value"=w139) -> ()  [unwired: 1 in, 2 out]
        n244 = call-poly <vilib>:"DAQmx Write.vi"("task/channels in"=w147, "data"=w137, "error in"=w144) -> ("task out"=w143:refnum<k21>, "error out"=w142:errorcluster)  [unwired: 10 in, 1 out]
        n245 = Build Array(w141, w134, w136) -> (w135:bool[])
        n246 = call-poly <vilib>:"DAQmx Write.vi"("task/channels in"=w154, "data"=w135, "error in"=w129) -> ("task out"=w153:refnum<k21>, "error out"=w151:errorcluster)  [unwired: 10 in, 1 out]
        n247 = Wait Until Next ms Multiple(millisecond multiple=u32 100) -> ()  [unwired: 1 out]
        n248 = property on="Salir" class="Bool (strict)"() -> ("Value"=w160:bool)  [unwired: 2 in, 2 out]
      }
      n249 = Current VI's Menubar() -> (w101:refnum<k9>)
      n250 = Delete Menu Items(9:w101) -> (3:w100:refnum<k9>)  [unwired: 3 in, 1 out]
      n251 = Insert Menu Items(8:string[] ["Calibra", "About"] ("item names"), 9:w100) -> (3:w99:refnum<k9>)  [unwired: 4 in, 2 out]
      n252 = while {
        tunnel: w99 -> [w162]
        stop <- w164 stop-if-true
        n253 = Get Menu Selection(0:w162, 1:200 ("ms timeout (200)")) -> (6:w161:string)  [unwired: 2 in, 4 out]
        n254 = case shown="\"Calibra\"" w161 {
          frame "False", Default {
          }
          frame "Calibra" {
            n255 = call "Calibra.vi"() -> ("SurtOk?"=w166:bool, "Factor Potència Out"=w165:dbl)  [unwired: 10 in]
            n256 = case shown="True" w166 {
              tunnel: w165 -> [_ w167]
              frame False {
              }
              frame True {
                n257 = control-ref of="mT1"() -> (w169:refnum<vi>)
                n258 = property on="Factor" class="DigNum (strict)"("Value"=w167) -> ()  [unwired: 2 in, 2 out]
                n259 = call "LecturaCal.vi"("T1"=w169) -> ("error out"=w168:errorcluster)  [unwired: 8 in, 2 out]
                n260 = case shown="Error" w168 {
                  frame No Error {
                    n261 = property on="mT1" class="DigNum (strict)"() -> ("Value"=w171:sgl)  [unwired: 2 in, 2 out]
                    n262 = Build Array(sgl 1.0 ("element"), w171) -> (w172:sgl[])
                    n263 = property on="PendentsT" class="Arr (strict)"("Value"=w172) -> ()  [unwired: 2 in, 2 out]
                  }
                  frame Error {
                  }
                }
              }
            }
          }
          frame "About" {
            n264 = call "About.vi"() -> ()  [unwired: 1 in]
          }
        }
        n265 = property on="Salir" class="Bool (strict)"() -> ("Value"=w164:bool)  [unwired: 2 in, 2 out]
      }
      n266 = Build Array(w47, w47, w47) -> (w46:bool[])
      n267 = call <vilib>:"DAQmx Stop Task.vi"("task/channels in"=w84, "error in"=w77) -> ("task out"=w83:refnum<k21>, "error out"=w82:errorcluster)  [unwired: 12 in]
      n268 = call-poly <vilib>:"DAQmx Write.vi"("task/channels in"=w40, "data"=0.0, "error in"=w39) -> ("task out"=w37:refnum<k21>, "error out"=w38:errorcluster)  [unwired: 10 in, 1 out]
      n269 = call-poly <vilib>:"DAQmx Write.vi"("task/channels in"=w44, "data"=w46, "error in"=w43) -> ("task out"=w42:refnum<k21>, "error out"=w41:errorcluster)  [unwired: 10 in, 1 out]
      n270 = call <vilib>:"DAQmx Clear Task.vi"("task in"=w83, "error in"=w82) -> ()  [unwired: 13 in, 1 out]
      n271 = call <vilib>:"DAQmx Stop Task.vi"("task/channels in"=w37, "error in"=w38) -> ("task out"=w68:refnum<k21>, "error out"=w67:errorcluster)  [unwired: 12 in]
      n272 = call <vilib>:"DAQmx Stop Task.vi"("task/channels in"=w42, "error in"=w41) -> ("task out"=w79:refnum<k21>, "error out"=w78:errorcluster)  [unwired: 12 in]
      n273 = call <vilib>:"DAQmx Clear Task.vi"("task in"=w68, "error in"=w67) -> ()  [unwired: 13 in, 1 out]
      n274 = call <vilib>:"DAQmx Clear Task.vi"("task in"=w79, "error in"=w78) -> ()  [unwired: 13 in, 1 out]
    }
  }
